vi "test vim.vi"() -> ()   [LabVIEW 2020]
uses:
  <vilib>/Utility/miscctls.llb/LVPositionTypeDef.ctl
  <vilib>/Utility/traverseref.llb/TRef TravTarget.ctl
  8109de0a-c5e5-4df9-99c1-24403cc15c95.vi
  <userlib>/_NEVSTOP/Communicable State Machine(CSM)/addons/MassData-Parameter/_support/FGV-MassData.vi
  CSM-Helper.lvclass
panel:
  out "Array 4":variant[](array[variant])
  out "Position":T1
  out "Array":string[](array[string])
  out "Label.Text":string
  out "Found?":bool
  in  "Include Instance VIs? (F)":bool
  out "# of SubVIs":i32
  out "SubVI Names":string[](array[string])
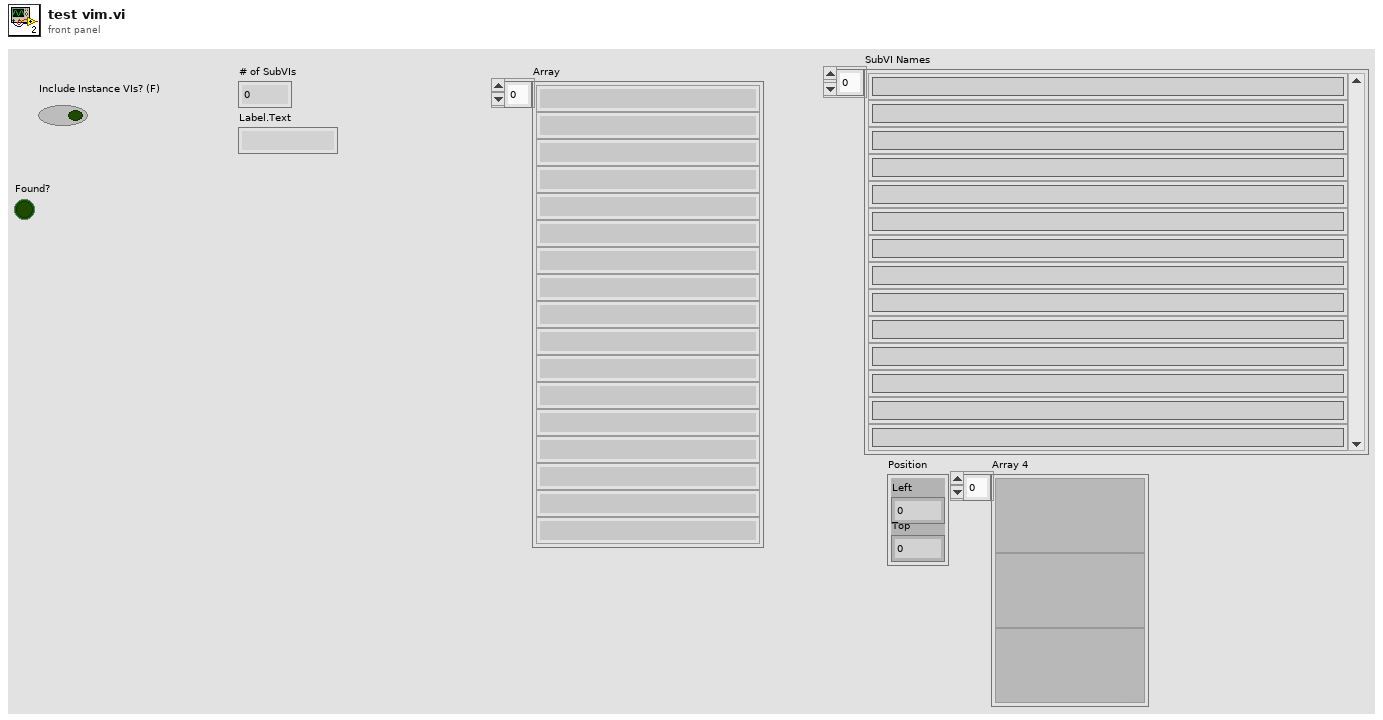
[diagram p1: front panel]
types:
  T1 = typedef "LVPositionTypeDef.ctl" = cluster{"Left":i32, "Top":i32}
  T2 = typedef "TRef TravTarget.ctl" = enum16{"FP", "BD", "Other"}
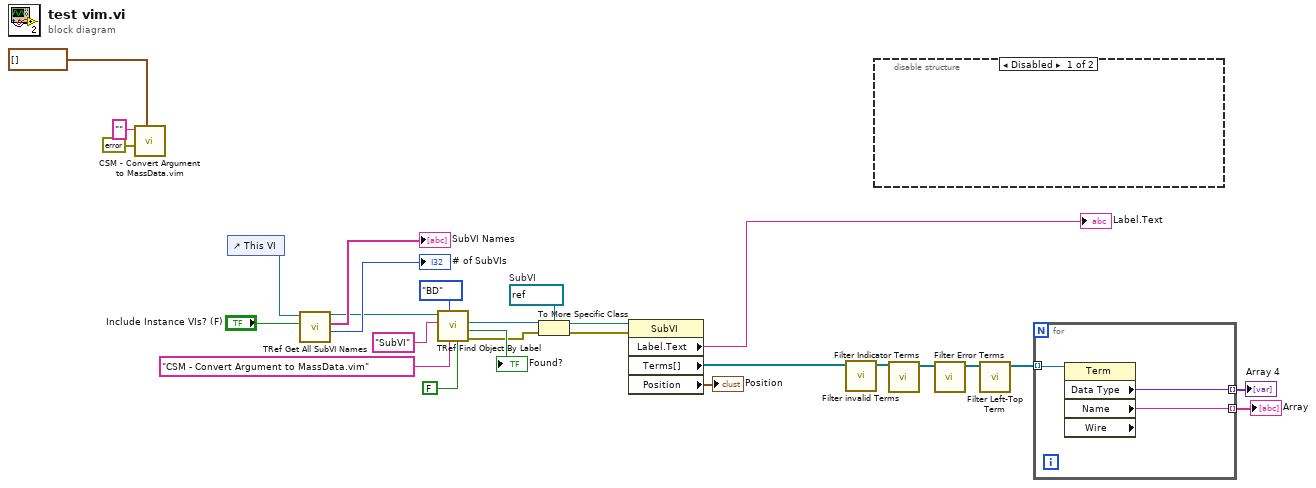
[diagram p0: block diagram]
diagram:
  w17 = refnum<vi> refnum  # SubVI
  n1 = call "CSM - Convert Argument to MassData.vim"("Type"=waveform(dbl)[] [] ("Data"), "error in (no error)"=errorcluster {"status"=FALSE, "code"=0, "source"=""}, "MassData Argument"="" ("String")) -> ()  [unwired: 5 in, 2 out]
  n2 = control-ref of="This VI"() -> (w27:refnum<vi>)
  n3 = call <vilib>:"TRef Get All SubVI Names.vi"("Include Instance VIs? (F)"="Include Instance VIs? (F)", "VI Refnum"=w27) -> ("# of SubVIs"=→"# of SubVIs":i32, "SubVI Names"=→"SubVI Names":string[], "dup VI Refnum"=w23:refnum<vi>)  [unwired: 5 in, 2 out]
  n4 = call <vilib>:"TRef Find Object By Label.vi"("Use Caption on Ctl? (F)"=FALSE, "Label"="CSM - Convert Argument to MassData.vim", "Traverse Target"=TRef_TravTarget."BD", "Class Name"="SubVI", "VI Ref"=w23) -> ("error out"=w16:errorcluster, "Found?"=→"Found?":bool, "Found Obj Ref"=w18:refnum<vi>)  [unwired: 3 in, 1 out]
  n5 = To More Specific Class(target class=w17, reference=w18, error in=w16) -> (specific class reference=w14:refnum<vi>, error out=w15:errorcluster)
  n6 = property class="SubVI"(reference=w14, error in=w15) -> ("Label.Text"=→"Label.Text":string, "Terms[]"=w7:refnum<vi>[], "Position"=→"Position":T1)  [unwired: 2 out]
  n7 = call "Filter invalid Terms.vi"("Terms[]"=w7) -> ("Terms[] out"=w6:refnum<vi>[])  [unwired: 10 in]
  n8 = disable-structure shown="Disabled" {
    frame Disabled {
    }
    frame Enabled {
    }
  }
  n9 = call "Filter Indicator Terms.vi"("Terms[]"=w6) -> ("Terms[] out"=w8:refnum<vi>[])  [unwired: 10 in]
  n10 = call "Filter Error Terms.vi"("Terms[]"=w8) -> ("Terms[] out"=w2:refnum<vi>[])  [unwired: 10 in]
  n11 = call "Filter Left-Top Term.vi"("Terms[]"=w2) -> ("Terms[] out"=w1:refnum<vi>[])  [unwired: 10 in]
  n12 = for {
    tunnel: w1 -> [w30] mode=indexing
    tunnel: [w29] -> w4 mode=indexing
    tunnel: [w28] -> w3 mode=indexing
    n13 = property class="Term" props=["Data Type", "Name", "Wire"](reference=w30) -> ("Data Type"=w28:variant, "Name"=w29:string)  [unwired: 1 in, 3 out]
  }
  "Array" <- w4
  "Array 4" <- w3
